vi "Persistent Data Menu.vi"() -> ()   [LabVIEW 2013]
panel:
  in  "File Name Prefix":string
  in  "Save Directory":path
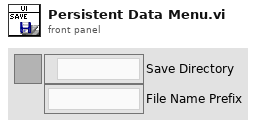
[diagram p1: front panel]
types:
  T1 = typedef "Semaphore RefNum" = refnum<k1>
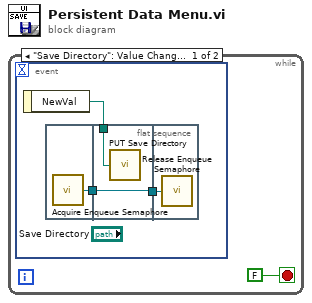
[diagram p0: block diagram]
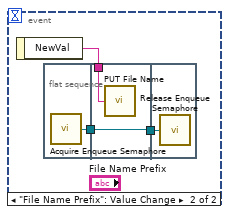
[diagram p2: hidden frame]
diagram:
  n1 = while {
    stop <- FALSE stop-if-true
    n2 = event shown="[0] \"Save Directory\": Value Change" {
      selector: _ -> [_ _]
      dyn-events: _ -> [_ _]
      timeout: _ -> [_ _]
      event "Save Directory": Value Change {
        n3 = event-data() -> ("NewVal"=w2:path)  [unwired: 1 in]
        n4 = flat-sequence {
          tunnel: [w5] -> w4
          tunnel: w4 -> [w7]
          tunnel: [w7] -> w3
          tunnel: w2 -> [w6]
          tunnel: w3 -> [w8]
          frame #0 {
            n5 = call "Acquire Enqueue Semaphore.vi"() -> ("Semaphore Reference"=w5:T1)
          }
          frame #1 {
            n6 = call "PUT Save Directory.vi"("Save Directory"=w6) -> ()
          }
          frame #2 {
            n7 = call "Release Enqueue Semaphore.vi"("Semaphore Reference"=w8) -> ()
          }
        }
      }
      event "File Name Prefix": Value Change {
        n8 = event-data() -> ("NewVal"=w9:string)  [unwired: 1 in]
        n9 = flat-sequence {
          tunnel: [w12] -> w11
          tunnel: w11 -> [w14]
          tunnel: [w14] -> w10
          tunnel: w9 -> [w13]
          tunnel: w10 -> [w15]
          frame #0 {
            n10 = call "Acquire Enqueue Semaphore.vi"() -> ("Semaphore Reference"=w12:T1)
          }
          frame #1 {
            n11 = call "PUT File Name.vi"("File Name"=w13) -> ()
          }
          frame #2 {
            n12 = call "Release Enqueue Semaphore.vi"("Semaphore Reference"=w15) -> ()
          }
        }
      }
    }
  }
